vi "GetPeakPositionByGaussCenter.vi"(11 "Input cluster":cluster{dbl[], dbl[]}) -> (0 "Gauss center position [mm]":dbl, 1 "Best Gaussian Fit":dbl[](array[numeric]), 2 "Peak amplitudes":dbl[](array[numeric]), 3 "Peak locations":dbl[](array[numeric]), 4 "Gauss residue":dbl)   [LabVIEW 2013]
uses:
  <vilib>/Analysis/6fits.llb/Curve Fitting Criteria.ctl
  <vilib>/Analysis/NI_AALPro.lvlib
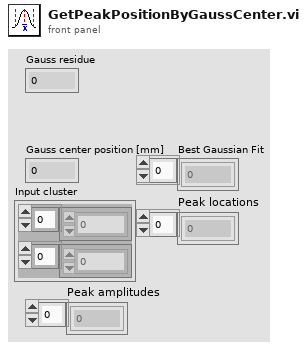
[diagram p1: front panel]
types:
  T1 = cluster{"initial amplitude":dbl, "initial center":dbl, "initial standard deviation":dbl, "offset":dbl}
  T2 = typedef "NI_AALPro.lvlib/Curve Fitting Criteria.ctl" = u16
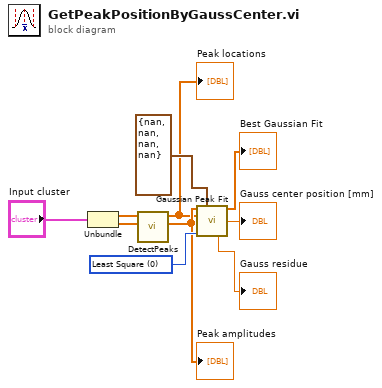
[diagram p0: block diagram]
diagram:
  w8 = T2 0 items=["Least Square", "Least Absolute Residual", "Bisquare"] ("method")
  n1 = Unbundle("Input cluster") -> (w2:dbl[], w5:dbl[])
  n2 = call "DetectPeaks.vi"("Y"=w5, "X"=w2) -> ("Amplitudes"=w7:dbl[], "Locations"=w1:dbl[])  [unwired: 8 in]
  "Peak locations" <- w1
  "Peak amplitudes" <- w7
  n3 = call <vilib>:"Gaussian Peak Fit.vi"("Y"=w7, "initial guess"=T1 {"initial amplitude"=nan, "initial center"=nan, "initial standard deviation"=nan, "offset"=nan}, "X"=w1, "method"=w8) -> ("Best Gaussian Fit"=→"Best Gaussian Fit":dbl[], "center"=→"Gauss center position [mm]":dbl, "residue"=→"Gauss residue":dbl)  [unwired: 5 in, 4 out]
